vi "Delta_counts2rad.vi"(11 "Numeric in":dbl) -> (3 "Numeric":dbl)   [LabVIEW 2019]
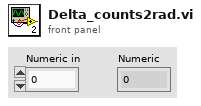
[diagram p1: front panel]
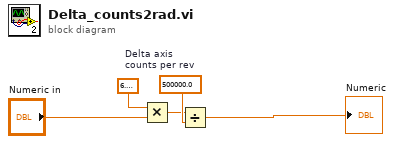
[diagram p0: block diagram]
diagram:
  w5 = 500000.0  # Delta axis  counts per rev
  n1 = Multiply(x=6.283185307179586, y="Numeric in") -> (x*y=w3:dbl)
  n2 = Divide(x=w3, y=w5) -> (x/y=→"Numeric":dbl)
